vi "Get Message.vi"(11 "error in (no error)":errorcluster) -> (4 "Message Type":T1, 8 "Data":variant, 15 "error out":errorcluster)   [LabVIEW 2016, in "Hall Effect Library.lvlib"]
doc: "This VI retreives a message from the Library's message queue. It returns the type of the message and it's corresponding data. Use the message type to determine which output contains valid data."
uses:
  Hall Effect Library.lvlib
  Controls/Message Types.ctl
  Private/Global Variables/Communication.vi
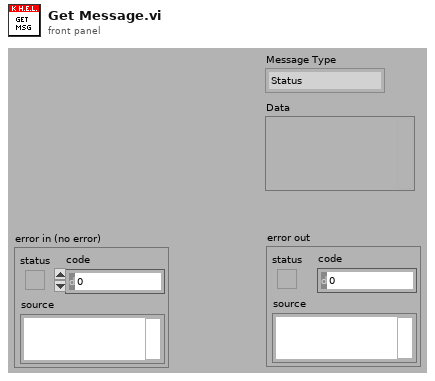
[diagram p1: front panel]
types:
  T1 = typedef "Hall Effect Library.lvlib/Message Types.ctl" = enum16{"Status", "New Data", "Test End Normal", "Test End User Abort", "Test End Error"}
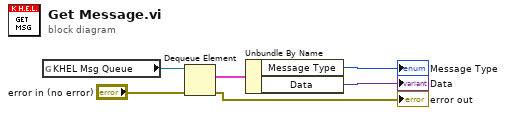
[diagram p0: block diagram]
diagram:
  n1 = global read "Communication.vi" "KHEL Msg Queue"() -> (w6:refnum<queue>)
  n2 = Dequeue Element(queue=w6, error in (no error)="error in (no error)") -> (element=w4:cluster{"Message Type":T1, "Data":variant}, error out=→"error out":errorcluster)  [unwired: 3 out]
  n3 = Unbundle By Name(w4) -> ("Message Type"=→"Message Type":T1, "Data"=→"Data":variant)
